vi "Check Target.vi"(8 "Error In":errorcluster, 9 "Target considered lost after frame":i32=3, 10 "Refocus threshold":dbl=0.125, 11 "Focus and Tracking":T1) -> (0 "Error out":errorcluster, 1 "CFS":dbl, 2 "Scope Error":bool, 3 "Target OK":bool, 4 "Optical Coordinates [um]":cluster{"X":dbl, "Y":dbl, "Z":dbl}, 5 "Need to refocus":bool, 7 "Area":dbl)   [LabVIEW 2012, in "Targeting Unit.lvlib"]
uses:
  Targeting Unit.lvlib
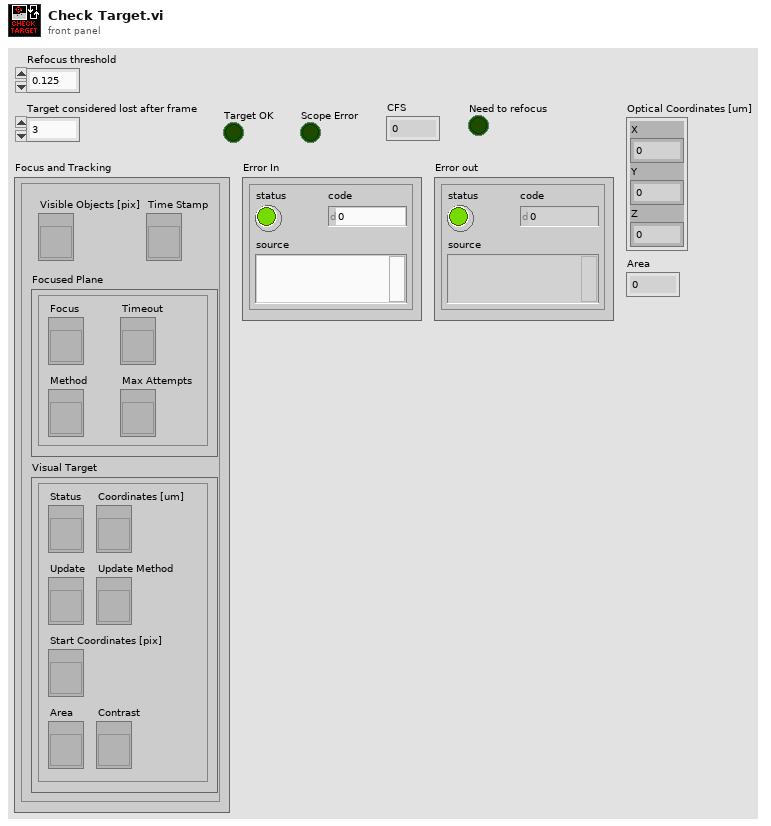
[diagram p1: front panel]
types:
  T1 = cluster{"Focused Plane":cluster{"Focus":refnum<vi>, "Timeout":refnum<vi>, "Max Attempts":refnum<vi>, "Method":refnum<vi>}, "Time Stamp":refnum<vi>, "Visual Target":cluster{"Coordinates [um]":refnum<vi>, "Status":refnum<vi>, "Update":refnum<vi>, "Update Method":refnum<vi>, "Start Coordinates [pix]":refnum<vi>, "Area":refnum<vi>, "Contrast":refnum<vi>}, "Visible Objects [pix]":refnum<vi>}
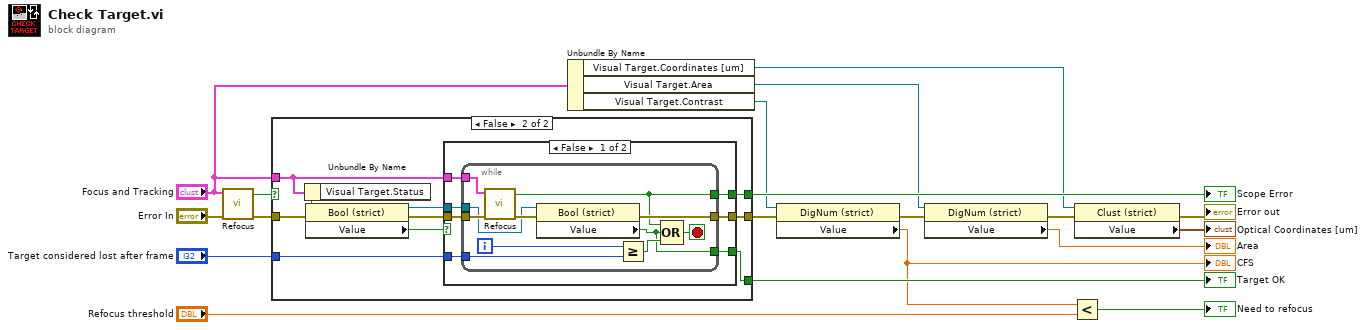
[diagram p0: block diagram]
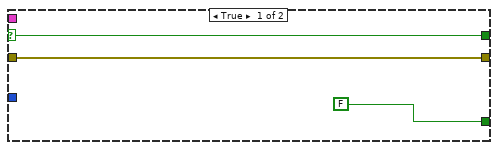
[diagram p2: hidden frame]
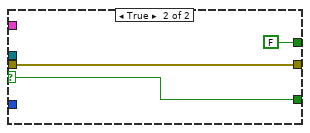
[diagram p3: hidden frame]
diagram:
  n1 = call "Refocus.vi"("Error In"="Error In", "Focus and Tracking"="Focus and Tracking") -> ("Error Out"=w18:errorcluster, "Error"=w17:bool)  [unwired: 8 in]
  n2 = case shown="False" w17 {
    selector: w17 -> [w20 _]
    tunnel: w18 -> [w21 w32]
    tunnel: "Focus and Tracking" -> [_ w24]
    tunnel: [FALSE w28] -> w16
    tunnel: [w21 w23] -> w13
    tunnel: "Target considered lost after frame" -> [_ w26]
    tunnel: [w20 w25] -> w14
    frame True {
    }
    frame False {
      n3 = Unbundle By Name(w24) -> ("Visual Target.Status"=w30:refnum<vi>)
      n4 = property class="Bool (strict)"(reference=w30, error in=w32) -> (reference out=w27:refnum<vi>, error out=w29:errorcluster, "Value"=w31:bool)
      n5 = case shown="False" w31 {
        selector: w31 -> [_ w53]
        tunnel: w29 -> [w39 w52]
        tunnel: w24 -> [w38 _]
        tunnel: [w35 w53] -> w28
        tunnel: [w36 w52] -> w23
        tunnel: w27 -> [w37 _]
        tunnel: w26 -> [w34 _]
        tunnel: [w33 FALSE ("Error")] -> w25
        frame False {
          n6 = while {
            tunnel: w39 -> [w50]
            tunnel: w38 -> [w49]
            tunnel: w37 -> [w46]
            tunnel: [w45] -> w36
            tunnel: [w40] -> w35
            tunnel: w34 -> [w44]
            tunnel: [w43] -> w33
            i -> [w48]
            stop <- w41 stop-if-true
            n7 = call "Refocus.vi"("Error In"=w50, "Focus and Tracking"=w49) -> ("Error Out"=w47:errorcluster, "Error"=w43:bool)  [unwired: 8 in]
            n8 = property class="Bool (strict)"(reference=w46, error in=w47) -> (error out=w45:errorcluster, "Value"=w40:bool)  [unwired: 1 out]
            n9 = Greater Or Equal?(x=w48, y=w44) -> (x >= y?=w42:bool)
            n10 = Compound Arithmetic op=OR(w43, w40, w42) -> (w41:bool)
          }
        }
        frame True {
        }
      }
    }
  }
  "Target OK" <- w16
  "Scope Error" <- w14
  n11 = Unbundle By Name("Focus and Tracking") -> ("Visual Target.Coordinates [um]"=w5:refnum<vi>, "Visual Target.Area"=w2:refnum<vi>, "Visual Target.Contrast"=w11:refnum<vi>)
  n12 = property class="DigNum (strict)"(reference=w11, error in=w13) -> (error out=w4:errorcluster, "Value"=w8:dbl)  [unwired: 1 out]
  "CFS" <- w8
  n13 = property class="DigNum (strict)"(reference=w2, error in=w4) -> (error out=w3:errorcluster, "Value"=→"Area":dbl)  [unwired: 1 out]
  n14 = Less?(x=w8, y="Refocus threshold") -> (x < y?=→"Need to refocus":bool)
  n15 = property class="Clust (strict)"(reference=w5, error in=w3) -> (error out=→"Error out":errorcluster, "Value"=→"Optical Coordinates [um]":cluster{"X":dbl, "Y":dbl, "Z":dbl})  [unwired: 1 out]
